vi "String If.vi"(7 "String In":string, 10 "If":bool) -> (2 "String":string)   [LabVIEW 2020, in "Promises.lvlib" / "Future.lvclass"]
uses:
  Future.lvclass
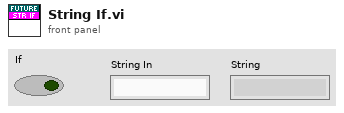
[diagram p1: front panel]
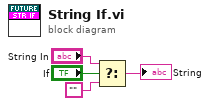
[diagram p0: block diagram]
diagram:
  n1 = Select(t="String In", s="If", f="") -> (s? t:f=→"String":string)
